vi "abbrevDetectorName.vi"(8 "error in":errorcluster, 11 "Canonical Name":string) -> (0 "error out":errorcluster, 3 "Abbreviated Detector Name":string)   [LabVIEW 2016]
doc: "Abbreviate the canonical detector name (e.g. \"R:2,2 S:1,1\" to \"R22_S11\")."
uses:
  <vilib>/regexp/Match Regular Expression.xnode
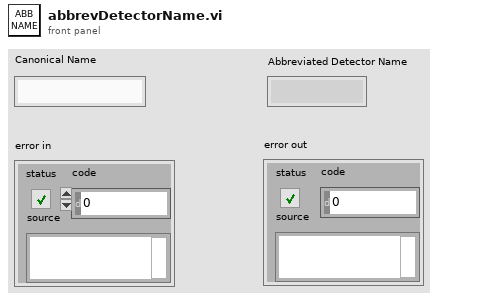
[diagram p1: front panel]
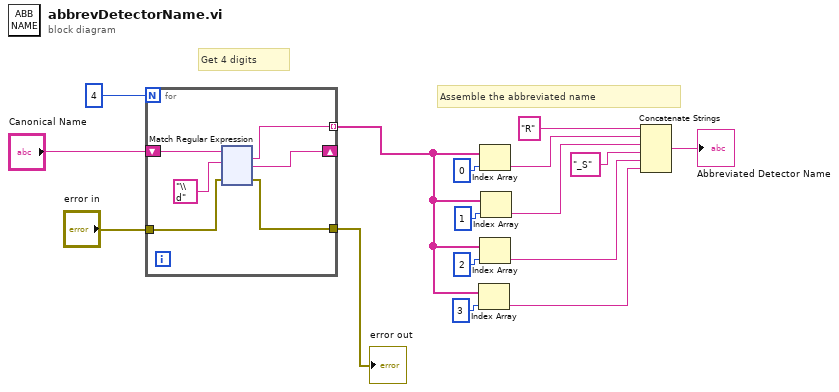
[diagram p0: block diagram]
diagram:
  # "Assemble the abbreviated name"
  # "Get 4 digits"
  n1 = for {
    N: 4 -> [_]
    shift-right: [w20] -> _
    shift-left: "Canonical Name" -> [w22]
    tunnel: [w19] -> w10 mode=indexing
    tunnel: "error in" -> [w18]
    tunnel: [w17] -> w14
    n2 = xnode "Match Regular Expression"("input string"=w22, "regular expression"="\\d", "error in"=w18) -> ("whole match"=w19:string, "after match"=w20:string, "error out"=w17:errorcluster)  [unwired: 3 in, 2 out]
  }
  "error out" <- w14
  n3 = Index Array(array=w10, index=3) -> (element=w2:string)
  n4 = Index Array(array=w10, index=0) -> (element=w6:string)
  n5 = Index Array(array=w10, index=2) -> (element=w3:string)
  n6 = Index Array(array=w10, index=1) -> (element=w5:string)
  n7 = Concatenate Strings("R" ("string"), w6, w5, "_S" ("string"), w3, w2) -> (→"Abbreviated Detector Name":string)
